vi "Create LUT Ref.vi"(8 "error in (no error)":errorcluster) -> (0 "error out":errorcluster, 3 "LUT out":refnum<class "LUT.lvclass">)   [LabVIEW 2017, in "LUT.lvlib" / "LUT.lvclass"]
doc: "Creates reference to the look up table (LUT).\nWe use LabVIEW Variant to create the LUT. The variant attributes are used to store name-data pairs."
uses:
  LUT.lvclass
  LUT.lvclass/LUT.ctl
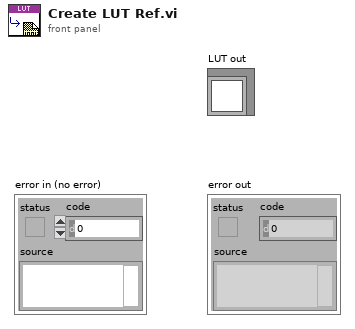
[diagram p1: front panel]
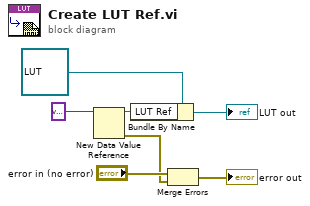
[diagram p0: block diagram]
diagram:
  n1 = New Data Value Reference(data value=variant) -> (data value reference=w6:refnum<data-value>, error out=w1:errorcluster)  [unwired: 1 in]
  n2 = Bundle By Name(cluster=refnum<class "LUT.lvclass"> refnum ("LUT.lvlib:LUT.lvclass"), "LUT Ref"=w6) -> (→"LUT out":refnum<class "LUT.lvclass">)
  n3 = Merge Errors("error in (no error)", w1) -> (→"error out":errorcluster)
